vi "prova.vi"() -> ()   [LabVIEW 2012]
uses:
  Debug/LabTIFF.dll
panel:
  out "size(s)":i32
  out "ErrorType 3":i32
  out "return type":i32
  in  "path":string
  in  "OpeningPurpose":string
  out "ErrorType 2":i32
  out "ErrorType":i32
  out "FileRef":i32
  out "error out":errorcluster
  out "Status 2":i32
  out "Status":i32
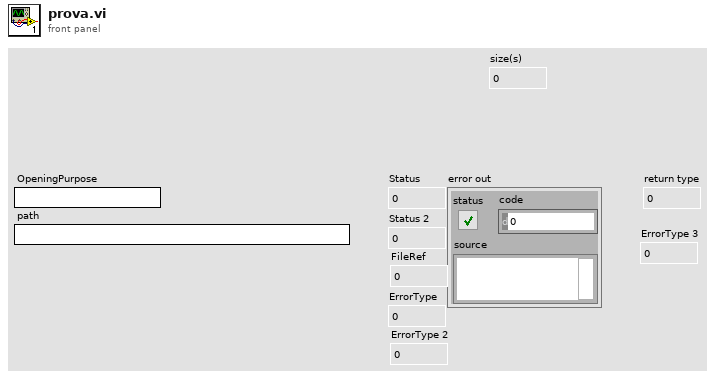
[diagram p1: front panel]
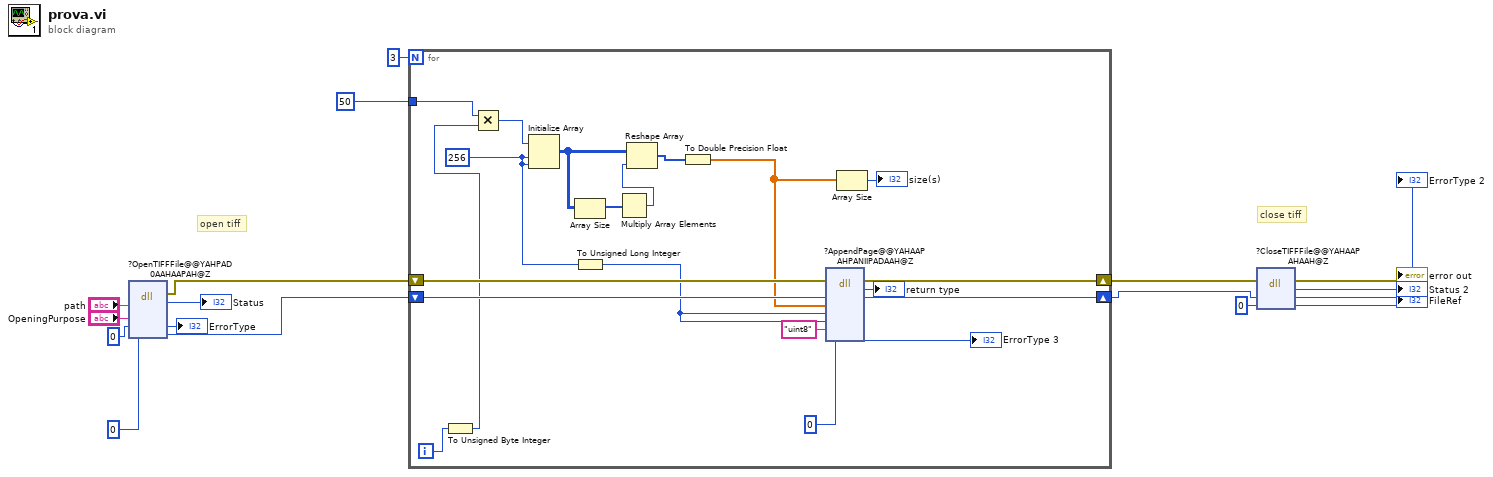
[diagram p0: block diagram]
diagram:
  # "close tiff"
  # "open tiff"
  n1 = dll-call lib="C:/Users/Ludo/Programming/Tests/TIFFManagement_test/LabTIFF/VisualCPP/LabTIFF/Debug/LabTIFF.dll" fn="?OpenTIFFFile@@YAHPAD0AAHAAPAH@Z"("path"="path", "OpeningPurpose"="OpeningPurpose", "ErrorType"=0, "FileRef"=0 ("ErrorType")) -> (error out=w7:errorcluster, "Status"=→"Status":i32, "ErrorType"=→"ErrorType":i32, "FileRef"=w15:i32)  [unwired: 5 in, 1 out]
  n2 = for {
    N: 3 -> [_]
    tunnel: u8 50 ("element") -> [w19]
    shift-right: [w27] -> w1
    shift-left: w7 -> [w36]
    shift-right: [w26] -> w2
    shift-left: w15 -> [w37]
    i -> [w21]
    w35 = 256 ("dimension size")
    n3 = To Unsigned Byte Integer(number=w21) -> (unsigned 8bit integer=w20:u8)
    n4 = Multiply(x=w19, y=w20) -> (x*y=w18:u8)
    n5 = Initialize Array(w18, w35, w35) -> (w30:u8[][])
    n6 = Array Size(array=w30) -> (size(s)=w29:i32[])
    n7 = To Unsigned Long Integer(number=w35) -> (unsigned 32bit integer=w34:u32)
    n8 = Multiply Array Elements(1:w29) -> (0:w28:i32)
    n9 = Reshape Array(w30, w28) -> (w33:u8[])
    n10 = To Double Precision Float(number=w33) -> (double precision float=w32:dbl[])
    n11 = dll-call lib="C:/Users/Ludo/Programming/Tests/TIFFManagement_test/LabTIFF/VisualCPP/LabTIFF/Debug/LabTIFF.dll" fn="?AppendPage@@YAHAAPAHPANIIPADAAH@Z"(error in=w36, "FileRef"=w37, "DataArray"=w32, "ImageHeight"=w34, "ImageWidth"=w34, "ImageType"="uint8", "ErrorType"=0) -> (error out=w27:errorcluster, "return type"=→"return type":i32, "FileRef"=w26:i32, "ErrorType"=→"ErrorType 3":i32)  [unwired: 6 in, 1 out]
    n12 = Array Size(array=w32) -> (size(s)=→"size(s)":i32)
  }
  n13 = dll-call lib="C:/Users/Ludo/Programming/Tests/TIFFManagement_test/LabTIFF/VisualCPP/LabTIFF/Debug/LabTIFF.dll" fn="?CloseTIFFFile@@YAHAAPAHAAH@Z"(error in=w1, "FileRef"=w2, "ErrorType"=0) -> (error out=→"error out":errorcluster, "Status"=→"Status 2":i32, "FileRef"=→"FileRef":i32, "ErrorType"=→"ErrorType 2":i32)  [unwired: 2 in, 1 out]
